vi "Begin.vi"(8 "error in":errorcluster) -> (0 "error out":errorcluster)   [LabVIEW 2019]
doc: "Called before other user functions, this VI is expected to open initial I/O refnums, load in file data, and do all program initialization. Notice that the <B>error out</B> terminal is simply used for data flow. Wiring it to other structures or subVIs ensures that this VI runs first."
uses:
  <vilib>/Rock Robotics/WPI/DriverStation/WPI_DriverStationRobotMode2.ctl
  Classes/Configuration File/Configuration File.lvclass
  TypeDefs/RobotObjects.ctl
  Classes/Drive/Tank Drive/Tank Drive.lvclass
  Classes/Pnematics control/Pneumatics.lvclass
  Classes/Vision/Vision.lvclass
  Classes/Joysticks/Joysticks.lvclass
  Classes/Elevator/Elevator.lvclass
  Classes/Hatch/Hatch.lvclass
  Classes/Cargo/Cargo.lvclass
  Classes/DriveOld/Drive.lvclass
  Classes/Robot/Robot.lvclass
  Classes/Control Panel/Control Panel.lvclass
  Classes/Climber/Climber.lvclass
  Classes/Turret/Turret.lvclass
  Classes/PowerCellHandler/Power Cell Handler.lvclass
  Classes/Joysticks/Joysticks.lvclass/Joysticks.ctl
  Classes/Joysticks/Public Methods/Write Sensitivity(x).vi
  Classes/Joysticks/Public Methods/Write Sensitivity(y).vi
  Robot Global Data.vi
  RobotGlobal.vi
  Classes/Drive/Tank Drive/CTRE Drive/CTRE Drive.lvclass
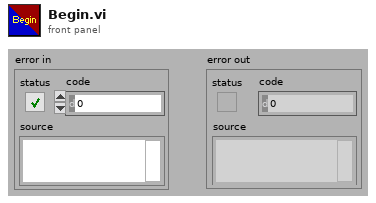
[diagram p1: front panel]
types:
  T1 = typedef "WPI_DriverStationRobotMode2.ctl" = enum16{"Autonomous Disabled", "Autonomous Enabled", "Teleop Disabled", "Teleop Enabled", "Disconnected", "Finish", "Test Disabled", "Test Enabled", "Emergency Stopped"}
  T2 = typedef "RobotObjects.ctl" = cluster{"Drive.lvclass":refnum<class "Tank Drive.lvclass">, "Pneumatics.lvclass":refnum<class "Pneumatics.lvclass">, "Vision.lvclass":refnum<class "Vision.lvclass">, "Joysticks.lvclass":refnum<class "Joysticks.lvclass">, "Elevator.lvclass":refnum<class "Elevator.lvclass">, "Hatch.lvclass":refnum<class "Hatch.lvclass">, "Cargo.lvclass":refnum<class "Cargo.lvclass">, "DriveOld.lvclass":refnum<class "Drive.lvclass">, "Robot.lvclass":refnum<class "Robot.lvclass">, "Control Panel.lvclass":refnum<class "Control Panel.lvclass">, "Climber.lvclass":refnum<class "Climber.lvclass">, "Turret.lvlib:Turret.lvclass":refnum<class "Turret.lvclass">, "Power Cell Handler.lvclass":refnum<class "Power Cell Handler.lvclass">}
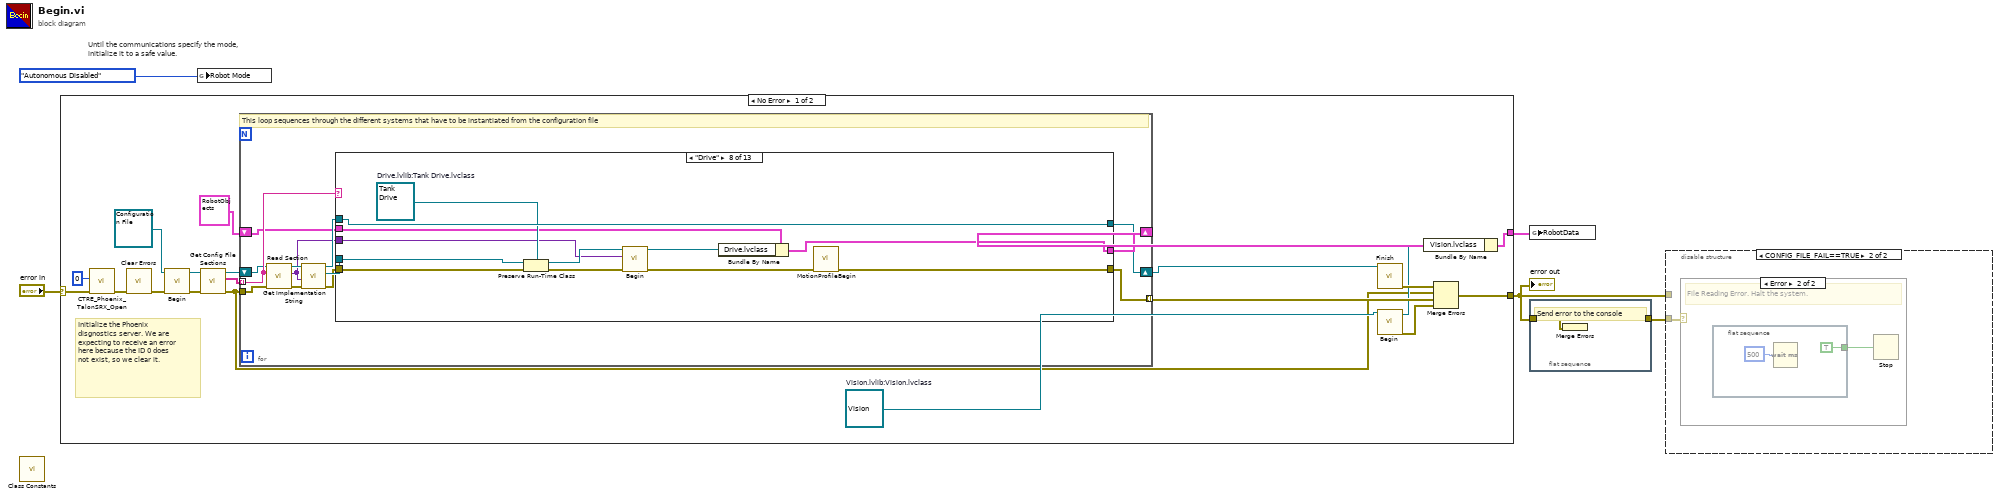
[diagram p0: block diagram]
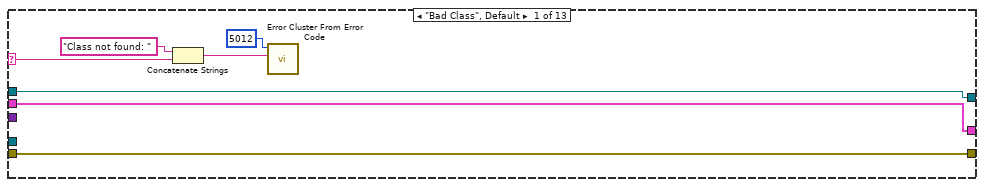
[diagram p2: hidden frame]
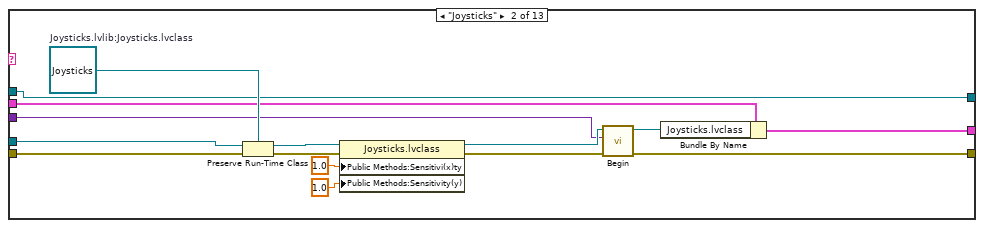
[diagram p3: hidden frame]
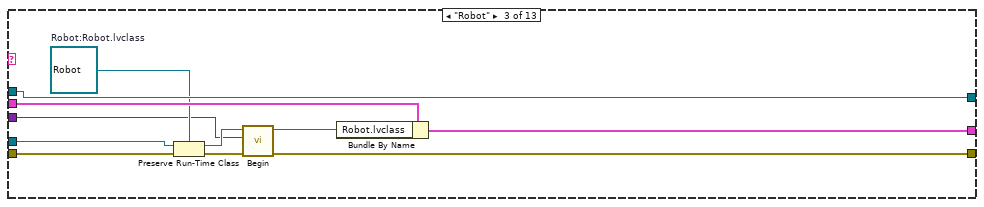
[diagram p4: hidden frame]
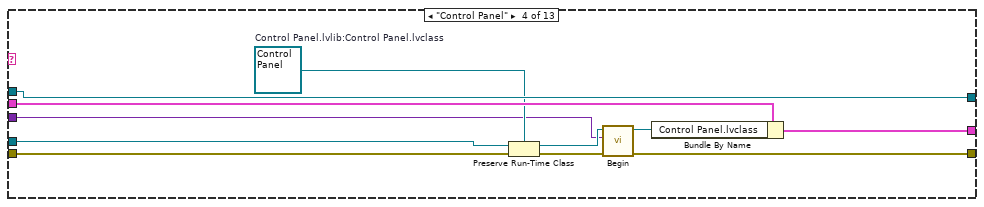
[diagram p5: hidden frame]
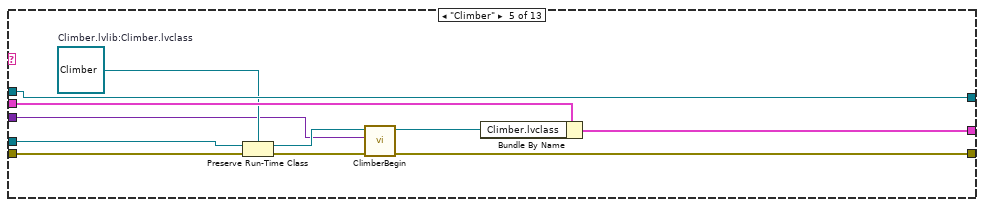
[diagram p6: hidden frame]
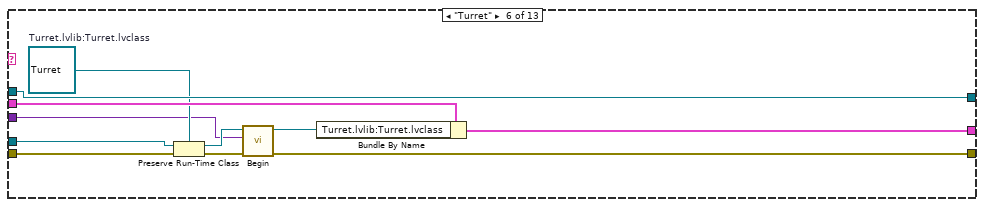
[diagram p7: hidden frame]
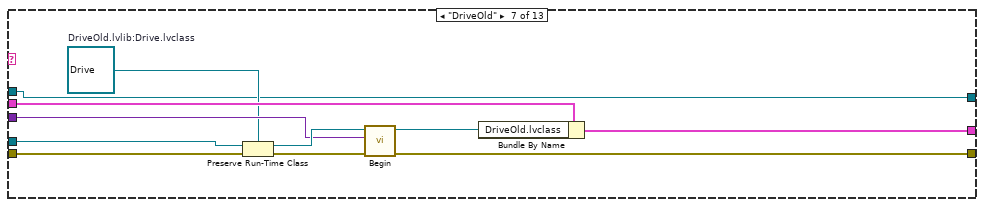
[diagram p8: hidden frame]
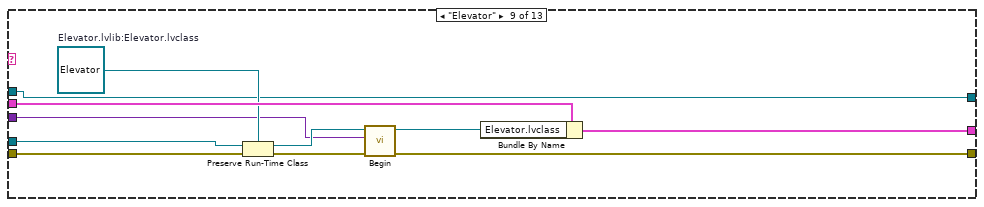
[diagram p9: hidden frame]
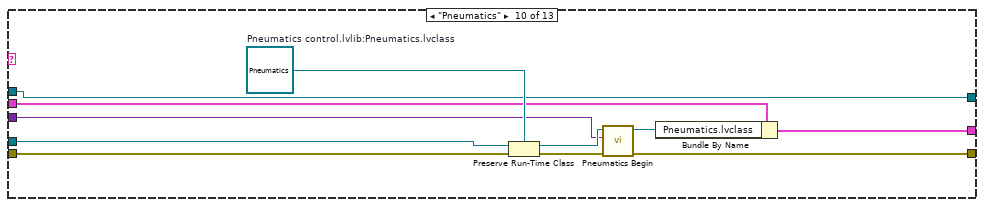
[diagram p10: hidden frame]
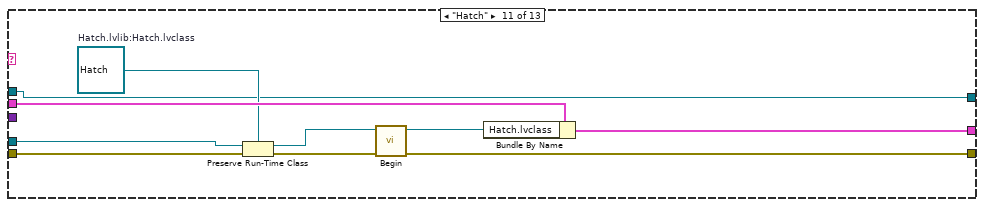
[diagram p11: hidden frame]
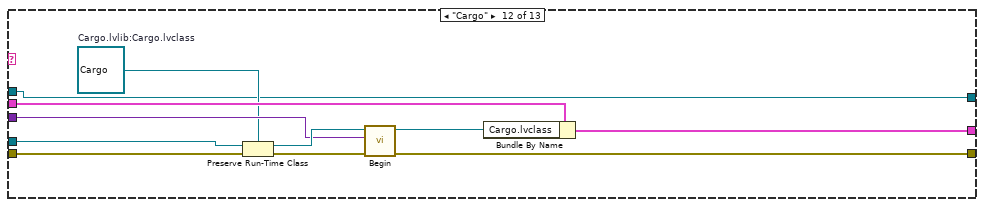
[diagram p12: hidden frame]
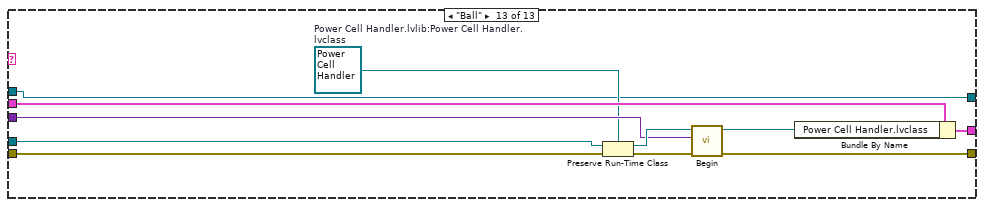
[diagram p13: hidden frame]
diagram:
  # "Until the communications specify the mode,\ninitialize it to a safe value."
  n1 = call "Class Constants.vi"() -> ()  [unwired: 12 in]
  n2 = case shown="No Error" "error in" {
    selector: "error in" -> [w22 w182]
    tunnel: [w16 _] -> w1
    tunnel: [w23 w182] -> w3
    frame No Error {
      w15 = refnum<class "Vision.lvclass"> refnum  # Vision.lvlib:Vision.lvclass
      # "Initialize the Phoenix disgnostics server. We are expecting to receive an error here because the ID 0 does not exist, so we clear it."
      n3 = call <vilib>:"CTRE_Phoenix_TalonSRX_Open.vi"("error in"=w22, "Device Number"=u8 0) -> ("error out"=w8:errorcluster)  [unwired: 8 in, 1 out]
      n4 = call <vilib>:"Clear Errors.vi"("error in (no error)"=w8) -> ("error out"=w6:errorcluster)  [unwired: 5 in, 1 out]
      n5 = call-dynamic "Begin.vi"("error in (no error)"=w6, "Configuration File in"=refnum<class "Configuration File.lvclass"> refnum) -> ("error out"=w19:errorcluster, "Configuration File out"=w11:refnum<class "Configuration File.lvclass">)  [unwired: 8 in]
      n6 = call-dynamic "Get Config File Sections.vi"("error in (no error)"=w19, "Configuration File in"=w11) -> ("error out"=w12:errorcluster, "Section names"=w9:string[], "Configuration File out"=w10:refnum<class "Configuration File.lvclass">)  [unwired: 7 in]
      n7 = for {
        tunnel: w9 -> [w38] mode=indexing
        tunnel: w12 -> [w27]
        shift-right: [w32] -> w21
        shift-left: T2 {"Drive.lvclass"=refnum, "Pneumatics.lvclass"=refnum, "Vision.lvclass"=refnum, "Joysticks.lvclass"=refnum, "Elevator.lvclass"=refnum, "Hatch.lvclass"=refnum, "Cargo.lvclass"=refnum, "DriveOld.lvclass"=refnum, "Robot.lvclass"=refnum, "Control Panel.lvclass"=refnum, "Climber.lvclass"=refnum, "Turret.lvlib:Turret.lvclass"=refnum, "Power Cell Handler.lvclass"=refnum} -> [w31]
        shift-right: [w29] -> w18
        shift-left: w10 -> [w30]
        tunnel: [w28] -> w17 mode=indexing
        # "This loop sequences through the different systems that have to be instantiated from the configuration file"
        n8 = call-dynamic "Read Section.vi"("error in (no error)"=w27, "Section Name"=w38, "Configuration File in"=w30) -> ("error out"=w36:errorcluster, "Data Out"=w34:variant, "Configuration File out"=w37:refnum<class "Configuration File.lvclass">)  [unwired: 5 in, 1 out]
        n9 = call-dynamic "Get Implementation String.vi"("error in (no error)"=w36, "Data In"=w34, "Configuration File in"=w37) -> ("error out"=w26:errorcluster, "Class Out"=w33:refnum<class>, "Configuration File out"=w35:refnum<class "Configuration File.lvclass">)  [unwired: 6 in]
        n10 = case shown="\"Drive\"" w38 {
          selector: w38 -> [w39 _ _ _ _ _ _ _ _ _ _ _ _]
          tunnel: w35 -> [w44 w46 w71 w82 w93 w104 w105 w127 w128 w140 w150 w160 w171]
          tunnel: w34 -> [_ w47 w61 w72 w83 w94 w107 w120 w129 w146 _ w162 w173]
          tunnel: w33 -> [_ w59 w67 w78 w89 w100 w115 w119 w138 w144 w159 w170 w181]
          tunnel: w26 -> [w43 w58 w69 w80 w91 w102 w114 w118 w137 w145 w158 w169 w180]
          tunnel: [w43 w57 w64 w75 w86 w97 w112 w116 w134 w147 w156 w166 w177] -> w28
          tunnel: [w45 w55 w62 w73 w84 w95 w110 w122 w132 w143 w154 w164 w175] -> w32
          tunnel: w31 -> [w45 w56 w70 w81 w92 w103 w111 w123 w133 w141 w155 w165 w176]
          tunnel: [w44 w46 w71 w82 w93 w104 w105 w127 w128 w140 w150 w160 w171] -> w29
          frame "Bad Class", Default {
            n11 = Concatenate Strings("Class not found: " ("error message (\"\")"), w39) -> (w40:string)
            n12 = call <vilib>:"Error Cluster From Error Code.vi"("error message (\"\")"=w40, "error code (0)"=5012) -> ()  [unwired: 7 in, 1 out]
          }
          frame "Joysticks" {
            w60 = refnum<class "Joysticks.lvclass"> refnum  # Joysticks.lvlib:Joysticks.lvclass
            n13 = Preserve Run-Time Class(object in=w59, error in=w58, 2:w60) -> (object out=w51:refnum<class "Joysticks.lvclass">, error out=w49:errorcluster)
            n14 = property class="Joysticks.lvclass"(reference=w51, error in=w49, "Public Methods:Sensitivi(x)ty"=1.0 ("Sensitivi(x)ty"), "Public Methods:Sensitivity(y)"=1.0 ("Sensitivity(y)")) -> (reference out=w50:refnum<class "Joysticks.lvclass">, error out=w48:errorcluster)
            n15 = call-dynamic "Begin.vi"("error in (no error)"=w48, "Settings In"=w47, "Joysticks in"=w50) -> ("error out"=w57:errorcluster, "Joysticks out"=w54:refnum<class "Joysticks.lvclass">)  [unwired: 7 in]
            n16 = Bundle By Name(cluster=w56, "Joysticks.lvclass"=w54) -> (w55:T2)
          }
          frame "Robot" {
            w68 = refnum<class "Robot.lvclass"> refnum  # Robot:Robot.lvclass
            n17 = Preserve Run-Time Class(object in=w67, error in=w69, 2:w68) -> (object out=w66:refnum<class "Robot.lvclass">, error out=w65:errorcluster)
            n18 = call-dynamic "Begin.vi"("error in (no error)"=w65, "variant in"=w61, "Robot in"=w66) -> ("error out"=w64:errorcluster, "Robot out"=w63:refnum<class "Robot.lvclass">)  [unwired: 7 in]
            n19 = Bundle By Name(cluster=w70, "Robot.lvclass"=w63) -> (w62:T2)
          }
          frame "Control Panel" {
            w79 = refnum<class "Control Panel.lvclass"> refnum  # Control Panel.lvlib:Control Panel.lvclass
            n20 = Preserve Run-Time Class(object in=w78, error in=w80, 2:w79) -> (object out=w77:refnum<class "Control Panel.lvclass">, error out=w76:errorcluster)
            n21 = call "Begin.vi"("error in (no error)"=w76, "Configuration In"=w72, "Control Panel in"=w77) -> ("error out"=w75:errorcluster, "Control Panel out"=w74:refnum<class "Control Panel.lvclass">)  [unwired: 7 in]
            n22 = Bundle By Name(cluster=w81, "Control Panel.lvclass"=w74) -> (w73:T2)
          }
          frame "Climber" {
            w90 = refnum<class "Climber.lvclass"> refnum  # Climber.lvlib:Climber.lvclass
            n23 = Preserve Run-Time Class(object in=w89, error in=w91, 2:w90) -> (object out=w88:refnum<class "Climber.lvclass">, error out=w87:errorcluster)
            n24 = call-dynamic "ClimberBegin.vi"("error in (no error)"=w87, "Configuration In"=w83, "Climber in"=w88) -> ("error out"=w86:errorcluster, "Climber out"=w85:refnum<class "Climber.lvclass">)  [unwired: 7 in]
            n25 = Bundle By Name(cluster=w92, "Climber.lvclass"=w85) -> (w84:T2)
          }
          frame "Turret" {
            w101 = refnum<class "Turret.lvclass"> refnum  # Turret.lvlib:Turret.lvclass
            n26 = Preserve Run-Time Class(object in=w100, error in=w102, 2:w101) -> (object out=w99:refnum<class "Turret.lvclass">, error out=w98:errorcluster)
            n27 = call "Begin.vi"("error in (no error)"=w98, "Config In"=w94, "Turret in"=w99) -> ("error out"=w97:errorcluster, "Turret out"=w96:refnum<class "Turret.lvclass">)  [unwired: 7 in]
            n28 = Bundle By Name(cluster=w103, "Turret.lvlib:Turret.lvclass"=w96) -> (w95:T2)
          }
          frame "DriveOld" {
            w106 = refnum<class "Drive.lvclass"> refnum  # DriveOld.lvlib:Drive.lvclass
            n29 = Preserve Run-Time Class(object in=w115, error in=w114, 2:w106) -> (object out=w108:refnum<class "Drive.lvclass">, error out=w113:errorcluster)
            n30 = call-dynamic "Begin.vi"("error in (no error)"=w113, "Settings"=w107, "Drive in"=w108) -> ("error out"=w112:errorcluster, "Drive out"=w109:refnum<class "Drive.lvclass">)  [unwired: 7 in]
            n31 = Bundle By Name(cluster=w111, "DriveOld.lvclass"=w109) -> (w110:T2)
          }
          frame "Drive" {
            w125 = refnum<class "Tank Drive.lvclass"> refnum  # Drive.lvlib:Tank Drive.lvclass
            n32 = Preserve Run-Time Class(object in=w119, error in=w118, 2:w125) -> (object out=w121:refnum<class "Tank Drive.lvclass">, error out=w126:errorcluster)
            n33 = call-dynamic "Begin.vi"("error in (no error)"=w126, "Config In"=w120, "Tank Drive in"=w121) -> ("error out"=w117:errorcluster, "Tank Drive out"=w124:refnum<class "Tank Drive.lvclass">)  [unwired: 7 in]
            n34 = Bundle By Name(cluster=w123, "Drive.lvclass"=w124) -> (w122:T2)
            n35 = call "MotionProfileBegin.vi"("error in (no error)"=w117) -> ("error out"=w116:errorcluster)  [unwired: 10 in]
          }
          frame "Elevator" {
            w130 = refnum<class "Elevator.lvclass"> refnum  # Elevator.lvlib:Elevator.lvclass
            n36 = Preserve Run-Time Class(object in=w138, error in=w137, 2:w130) -> (object out=w136:refnum<class "Elevator.lvclass">, error out=w135:errorcluster)
            n37 = call-dynamic "Begin.vi"("error in (no error)"=w135, "Settings"=w129, "Elevator in"=w136) -> ("error out"=w134:errorcluster, "Elevator out"=w131:refnum<class "Elevator.lvclass">)  [unwired: 7 in]
            n38 = Bundle By Name(cluster=w133, "Elevator.lvclass"=w131) -> (w132:T2)
          }
          frame "Pneumatics" {
            w149 = refnum<class "Pneumatics.lvclass"> refnum  # Pneumatics control.lvlib:Pneumatics.lvclass
            n39 = Preserve Run-Time Class(object in=w144, error in=w145, 2:w149) -> (object out=w148:refnum<class "Pneumatics.lvclass">, error out=w139:errorcluster)
            n40 = call "Pneumatics Begin.vi"("error in (no error)"=w139, "Data Out"=w146, "Pneumatics in"=w148) -> ("error out"=w147:errorcluster, "Pneumatics out"=w142:refnum<class "Pneumatics.lvclass">)  [unwired: 7 in]
            n41 = Bundle By Name(cluster=w141, "Pneumatics.lvclass"=w142) -> (w143:T2)
          }
          frame "Hatch" {
            w153 = refnum<class "Hatch.lvclass"> refnum  # Hatch.lvlib:Hatch.lvclass
            n42 = Preserve Run-Time Class(object in=w159, error in=w158, 2:w153) -> (object out=w152:refnum<class "Hatch.lvclass">, error out=w157:errorcluster)
            n43 = call-dynamic "Begin.vi"("error in (no error)"=w157, "Hatch in"=w152) -> ("error out"=w156:errorcluster, "Hatch out"=w151:refnum<class "Hatch.lvclass">)  [unwired: 8 in]
            n44 = Bundle By Name(cluster=w155, "Hatch.lvclass"=w151) -> (w154:T2)
          }
          frame "Cargo" {
            w161 = refnum<class "Cargo.lvclass"> refnum  # Cargo.lvlib:Cargo.lvclass
            n45 = Preserve Run-Time Class(object in=w170, error in=w169, 2:w161) -> (object out=w168:refnum<class "Cargo.lvclass">, error out=w167:errorcluster)
            n46 = call-dynamic "Begin.vi"("error in (no error)"=w167, "Configuration In"=w162, "Cargo in"=w168) -> ("error out"=w166:errorcluster, "Cargo out"=w163:refnum<class "Cargo.lvclass">)  [unwired: 7 in]
            n47 = Bundle By Name(cluster=w165, "Cargo.lvclass"=w163) -> (w164:T2)
          }
          frame "Ball" {
            w172 = refnum<class "Power Cell Handler.lvclass"> refnum  # Power Cell Handler.lvlib:Power Cell Handler.lvclass
            n48 = Preserve Run-Time Class(object in=w181, error in=w180, 2:w172) -> (object out=w179:refnum<class "Power Cell Handler.lvclass">, error out=w178:errorcluster)
            n49 = call "Begin.vi"("error in (no error)"=w178, "Configuration in"=w173, "Power Cell Handler in"=w179) -> ("error out"=w177:errorcluster, "Power Cell Handler out"=w174:refnum<class "Power Cell Handler.lvclass">)  [unwired: 7 in]
            n50 = Bundle By Name(cluster=w176, "Power Cell Handler.lvclass"=w174) -> (w175:T2)
          }
        }
      }
      n51 = call-dynamic "Finish.vi"("Configuration File in"=w18) -> ("error out"=w24:errorcluster)  [unwired: 7 in, 3 out]
      n52 = call-dynamic "Begin.vi"("Vision in"=w15) -> ("error out"=w13:errorcluster, "Vision out"=w14:refnum<class "Vision.lvclass">)  [unwired: 9 in]
      n53 = Bundle By Name(cluster=w21, "Vision.lvclass"=w14) -> (w16:T2)
      n54 = Merge Errors(w24, w12, w17, w13) -> (w23:errorcluster)
    }
    frame Error {
    }
  }
  "error out" <- w3
  n55 = global write "Robot Global Data.vi" "Robot Mode"(WPI_DriverStationRobotMode2."Autonomous Disabled" ("Robot Mode")) -> ()
  n56 = global write "RobotGlobal.vi" "RobotData"(w1) -> ()
  n57 = flat-sequence {
    tunnel: w3 -> [w183]
    tunnel: [w183] -> w2
    frame #0 {
      # "Send error to the console"
      n58 = Merge Errors(w183) -> ()  [unwired: 1 out]
    }
  }
  n59 = disable-structure shown="CONFIG_FILE_FAIL==TRUE" {
    disable-tunnel: w3 -> [_ _]
    disable-tunnel: w2 -> [_ w184]
    frame condition #0 (active) {
      # "If the project key to halt the execution if the configuration file is wrong\nis not activated, then do nothing if we have an error at the end."
    }
    frame condition #1 {
      n60 = case shown="Error" w184 {
        frame No Error {
        }
        frame Error {
          # "File Reading Error. Halt the system."
          n61 = flat-sequence {
            tunnel: [TRUE ("stop? (T)")] -> w185
            frame #0 {
              n62 = Wait (ms)(milliseconds to wait=u32 500) -> ()  [unwired: 1 out]
            }
          }
          n63 = Stop(stop? (T)=w185) -> ()
        }
      }
    }
  }
